vi "Congif TDMS file for multiple devices.vi"(6 "Queue in":refnum<queue>, 7 "HSS Resource references":refnum<k20>[](array[refnum]), 8 "error in (no error)":errorcluster, 9 "Playback Options":T1={"Infinite Generation"=FALSE, "max asynch. reads"=8, "Samples per Write"=1024000, "chunks"=16, "disable buffering?"=TRUE} {"chunks" format="%.0p"; "Samples per Write" format="%.3p"}, 10 "tx config":T3 {"sample rate" format="%#.3pS/s"; "rf config 0"."level" format="%#_gdBm"; "rf config 0"."lo frequency" format="%#.3pHz"; "rf config 0"."frequency" format="%#.3pHz"; "rf config 1"."level" format="%#_gdBm"; "rf config 1"."lo frequency" format="%#.3pHz"; "rf config 1"."frequency" format="%#.3pHz"}, 11 "TDMS controls in":T2[][](array[typedef])) -> (0 "error out":errorcluster, 3 "TDMS read controls out":T2[][](array[typedef]))   [LabVIEW 2016]
uses:
  TypeDefs/Tx Config.ctl
  2954/SubVIs/Start Trigger.ctl
  TypeDefs/TDMS read.ctl
  TypeDefs/Playback Options.ctl
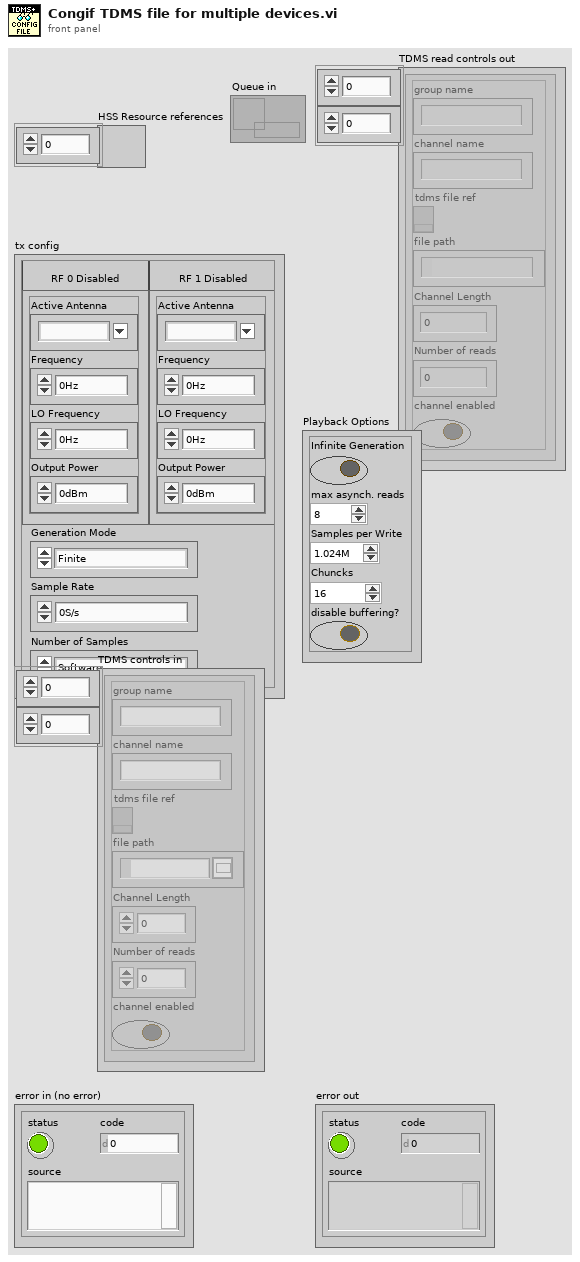
[diagram p1: front panel]
types:
  T1 = typedef "Playback Options.ctl" = cluster{"Infinite Generation":bool, "max asynch. reads":u32, "Samples per Write":u32, "chunks":u32, "disable buffering?":bool}
  T2 = typedef "TDMS read.ctl" = cluster{"group name":string, "channel name":string, "tdms file ref":refnum<k34>, "file path":path, "Channel Length":i64, "Number of reads":i64, "channel enabled":bool}
  T3 = typedef "Tx Config.ctl" = cluster{"rf enable 0":bool, "rf config 0":cluster{"antenna":string, "frequency":dbl, "lo frequency":dbl, "level":dbl}, "rf enable 1":bool, "rf config 1":cluster{"antenna":string, "frequency":dbl, "lo frequency":dbl, "level":dbl}, "transfer mode":enum16{"Finite", "Continuous"}, "sample rate":dbl, "start trigger":T4}
  T4 = typedef "Start Trigger.ctl" = enum8{"Software", "Digital Edge", "Rx Start Trigger", "Tx Start Trigger", "Immediate", "Future Time Event"}
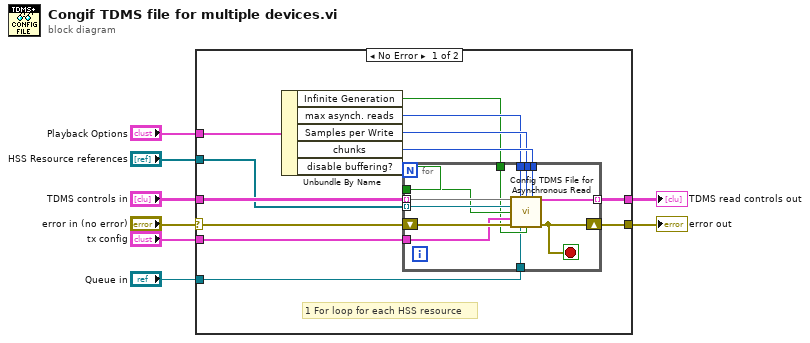
[diagram p0: block diagram]
diagram:
  n1 = case shown="No Error" "error in (no error)" {
    selector: "error in (no error)" -> [w16 w35]
    tunnel: "tx config" -> [w21 _]
    tunnel: "TDMS controls in" -> [w20 w34]
    tunnel: [w19 w34] -> w6
    tunnel: "HSS Resource references" -> [w18 _]
    tunnel: [w17 w35] -> w4
    tunnel: "Playback Options" -> [w15 _]
    tunnel: "Queue in" -> [w9 _]
    frame No Error {
      # "1 For loop for each HSS resource"
      n2 = Unbundle By Name(w15) -> ("Infinite Generation"=w10:bool, "max asynch. reads"=w12:u32, "Samples per Write"=w13:u32, "chunks"=w14:u32, "disable buffering?"=w11:bool)
      n3 = for {
        tunnel: w20 -> [w30] mode=indexing
        tunnel: w18 -> [w32] mode=indexing
        shift-right: [w23] -> w17
        shift-left: w16 -> [w33]
        tunnel: [w31] -> w19 mode=indexing
        tunnel: w21 -> [w29]
        tunnel: w14 -> [w28]
        tunnel: w13 -> [w27]
        tunnel: w12 -> [w26]
        tunnel: w11 -> [w25]
        tunnel: w10 -> [w24]
        tunnel: w9 -> [w22]
        stop <- w23 stop-if-true
        n4 = call "Config TDMS File for Asynchronous Read.vi"("TDMS read controls array"=w30, "max asynchronous reads"=w26, "Samples per Write"=w27, "chunks"=w28, "HSS refnum in"=w32, "disable buffering? (T)"=w25, "tx config"=w29, "error in (no error)"=w33, "Queue in"=w22, "Infinite Generation"=w24) -> ("TDMS read control array out"=w31:T2[], "error out"=w23:errorcluster)  [unwired: 2 in, 2 out]
      }
    }
    frame Error {
    }
  }
  "TDMS read controls out" <- w6
  "error out" <- w4
